vi "OCUMain.vi"() -> ()   [LabVIEW 2014]
uses:
  Command.ctl
  DataHighway.ctl
  <vilib>/Math Plots/2D Math Plots/2D Compass/2D Compass XCtrl/2D Compass.xctl
  MDF.ctl
  <vilib>/Math Plots/2D Math Plots/2D Compass/2D Compass Datatype/Public/Plot Helper (Vector).vi
  <vilib>/ErrorRing/Error Ring.xnode
  <vilib>/Math Plots/2D Math Plots/2D Compass/2D Compass Datatype/2D Compass Datatype.lvclass
panel:
  out "Tug GPS":cluster{"X pos":i32, "Y pos":i32, "Heading":dbl}
  out "UDP Time Out?":bool
  in  "Tug ?":string="T"
  out "Buoy Locations":cluster{"regular expression":string, i32, i32}[](array[cluster])
  out "GPS OK?":bool
  out "Mission Map In":picture
  in  "Stop OCU Code Running":bool
  in  "E-Stop Motors":bool=TRUE
  out "DataHWay":T1
  out "ComHWay":T2 {"Speed" scale=-2.0..10.0; "Rudder" scale=-10.0..10.0}
  out "OCU Running":bool
  out "Tab Control":T3(tab)
  out "PT Mid":dbl(slide) scale=60.0..20.0
  out "ST Mid":dbl(slide) scale=20.0..60.0
  out "ST Bow":dbl(slide) scale=20.0..60.0
  out "Starboard":dbl(slide) scale=20.0..60.0
  out "PT Bow":dbl(slide) scale=20.0..60.0
  out "Boolean 5":bool
  out "Boolean 4":bool
  out "Boolean 3":bool
  out "Boolean 2":bool
  out "Boolean":bool
  in  "Beh Lights ok?":bool
  in  "myRIO ok?":bool
  in  "Prop ok?":bool
  in  "Rudder ok?":bool
  in  "Sharp IR-Lidar ok?":bool
  in  "Goto Debug?":bool
  out "MyRIO":bool
  out "Port":dbl(slide) scale=60.0..20.0
  out "Tug GPS":cluster{"X pos":i32, "Y pos":i32, "Heading":dbl}
  out "Buoy locations":cluster{"regular expression":string, i32, i32}[](array[cluster])
  out "Waiting for Input":bool
  in  "Plan Mission":bool
  in  "Re-Initialize":bool
  in  "Debug Robot":bool
  in  "Run Robot":bool
  in  "Stop OCU":bool
  in  "Prop Speed":dbl(knob)=0.07590623483784206 scale=0.05..0.1
  in  "Rudder":dbl(knob)=0.0742658968653541 scale=0.05..0.1
  in  "Debug Complete?":bool
  out "RobotRunning":bool
  out "HW-Stop":bool
  out "IR LIDAR":refnum<class "2D Plot Datatype.lvclass">[](xcontrol)
  out "Tug GPS Debug":cluster{"X pos":i32, "Y pos":i32, "Heading":dbl}
  out "Buoy Locations Debug":cluster{"regular expression":string, i32, i32}[](array[cluster])
  in  "Exit Run":bool
  out "Tug GPS Run":cluster{"X pos":i32, "Y pos":i32, "Heading":dbl}
  out "Buoy Locations Run":cluster{"regular expression":string, i32, i32}[](array[cluster])
  out "Mission Map Run Robot":picture
  in  "Exit Planning":bool
  in  "Select Behavior":T4(ring)
  out "MDF":T5
  in  "Velocity":dbl(slide) scale=0.0..500.0
  in  "Dwell Time (sec)":dbl(slide) scale=0.0..10.0
  out "Draw Path":bool
  out "WPindex":i32
  in  "Reset MDF":bool
  out "Mission Map":picture
  # "Press Arrow\nabove to start\nOCU running"
  # "Set Tug\nLetter"
  # "G\nT\nL\n?"
  # "Data Highway carries all robot data"
  # "Look at boat. Rudder Oscillating?"
  # "Release E-Stop to test"
  # "Look at boat? Prop Oscillating?"
  # "Is battery attached?"
  # "Look at boat. See Red-Blue-Green?"
  # "Unit Test"
  # "Function"
  # "Run auto Initialize sequence.\nIndicate which functionality is ok.\nAll functions must work or\n choose go to debug state."
  # "Robot Initialized and \nwaiting for user input"
  # "Press button to\nselect robot state"
  # "0.075 rudder center"
  # "0.075 prop off"
  # "OCU and Robot safely shut down"
  # "2. Click on Map to select Waypoints, hold button down and drag to draw tracklines.\n3. Reset MDF and try again if you want to redo your MDF"
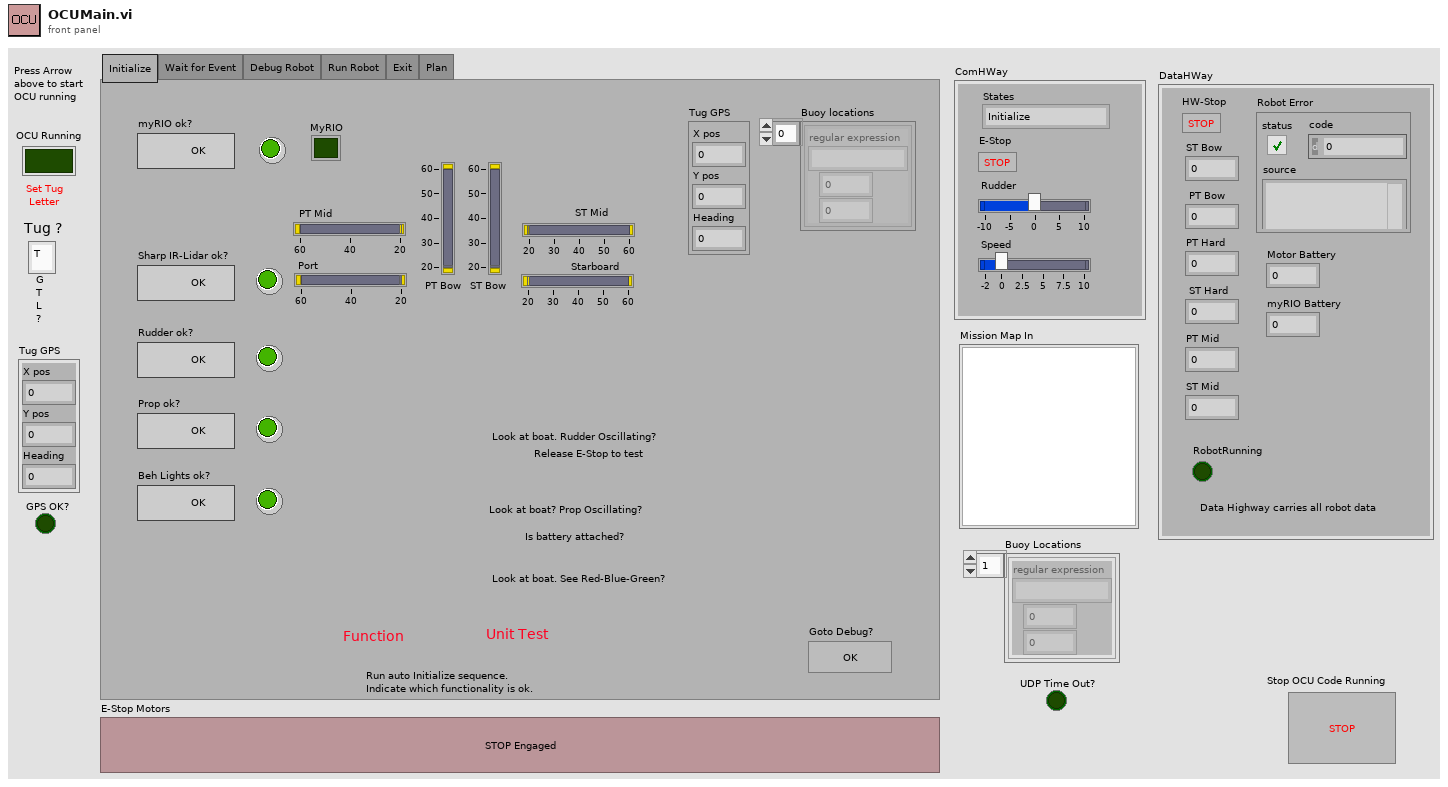
[diagram p1: front panel]
types:
  T1 = typedef "DataHighway.ctl" = cluster{"HW-Stop":bool, "ST Bow":dbl, " PT Bow":dbl, "PT Hard":dbl, "RobotRunning":bool, "Robot Error":errorcluster, " ST Hard":dbl, "PT Mid":dbl, "ST Mid":dbl, "Motor Battery":dbl, "myRIO Battery":dbl}
  T2 = typedef "Command.ctl" = cluster{"States":enum16{"Initialize", "Wait for Event", "Debug Robot", "Run Robot", "Exit", "Plan"}, "E-Stop":bool, "Rudder":dbl, "Speed":dbl}
  T3 = enum32{"Initialize", "Wait for Event", "Debug Robot", "Run Robot", "Exit", "Plan"}
  T4 = enum16{"Stop", "GoToWayPoint", "RightWallFollow", "LeftWallFolllow", "LaneFollow", "CirclePoint"}
  T5 = typedef "MDF.ctl" = cluster{"Status":enum16{"Past", "Current", "Future"}, "x":dbl, "y":dbl, "z":dbl, "Vel":dbl, "Dwell Time":dbl, "BehCom":enum16{"Stop", "GoToWayPoint", "RightWallFollow", "LeftWallFolllow", "LaneFollow", "CirclePoint"}, "Expand1":dbl, "Expand2":dbl, "Expand3":dbl}[]
  T6 = cluster{"Status":enum16{"Past", "Current", "Future"}, "x":dbl, "y":dbl, "z":dbl, "Vel":dbl, "Dwell Time":dbl, "BehCom":enum16{"Stop", "GoToWayPoint", "RightWallFollow", "LeftWallFolllow", "LaneFollow", "CirclePoint"}, "Expand1":dbl, "Expand2":dbl, "Expand3":dbl}
  T7 = enum16{"Initialize", "Wait for Event", "Debug Robot", "Run Robot", "Exit", "Plan"}
  T8 = enum16{"Initialize", "Wait for Event", "Debug Robot", "Run Robot", "Exit"}
  T9 = cluster{"Width":u16, "Style":enum32{"Solid", "Dash", "Dot", "DashDot", "DashDotDot"}}
  T10 = typedef "LVMouseTypeDef.ctl" = cluster{"Mouse Position":cluster{"X":i32, "Y":i32}, "Mouse Modifiers":cluster{"Button Down":bool, "Shift Mod":bool, "Menu Mod":bool, "Option Mod":bool}}
  T11 = cluster{"regular expression":string, i32, i32, i32}
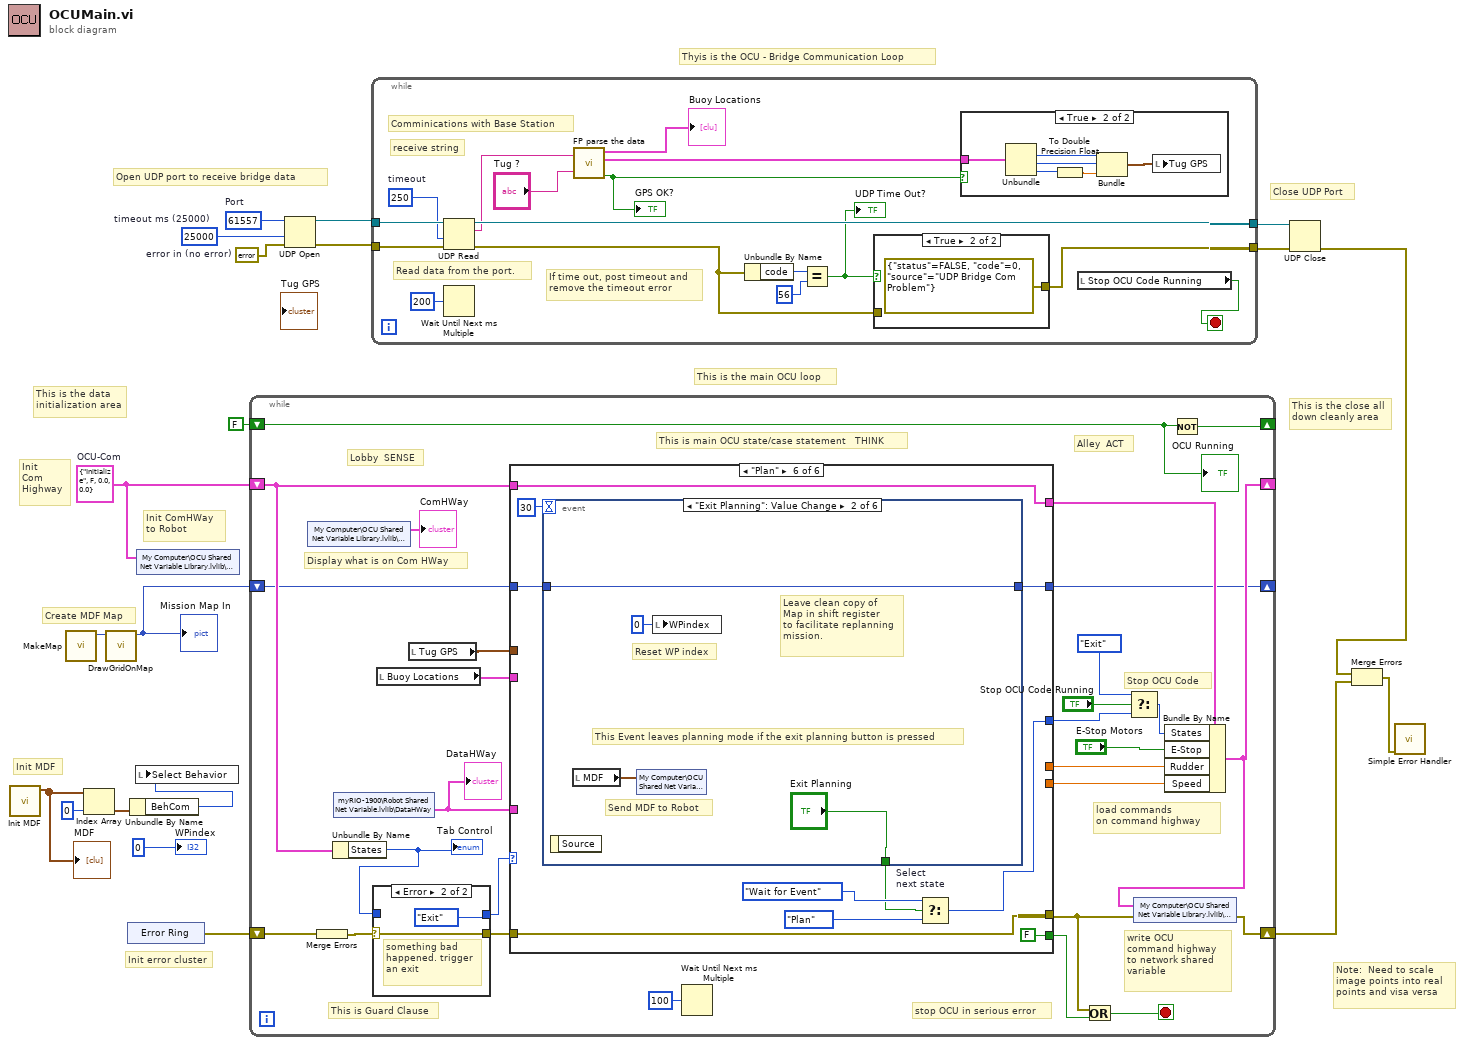
[diagram p0: block diagram]
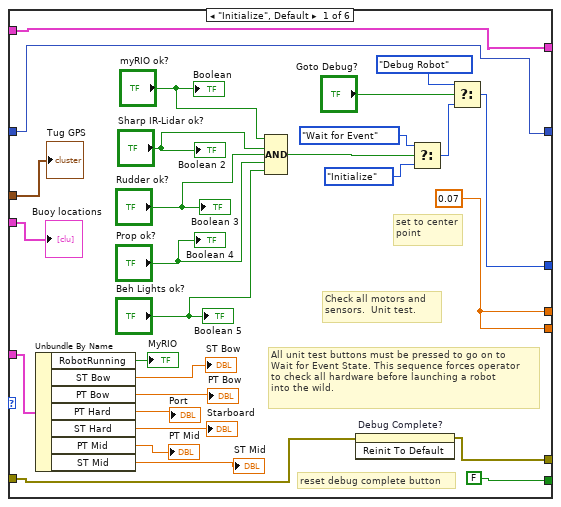
[diagram p5: hidden frame]
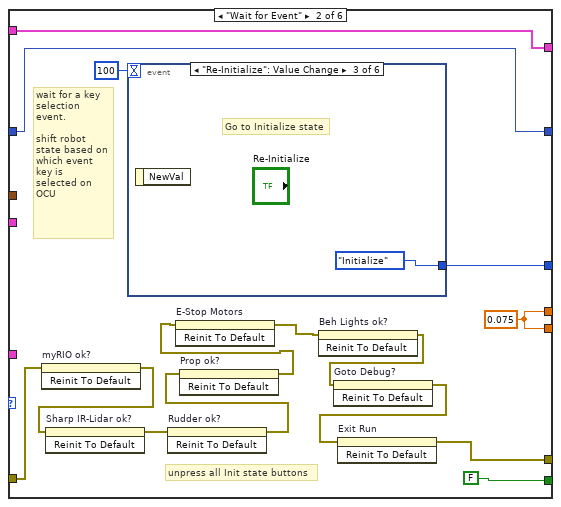
[diagram p6: hidden frame]
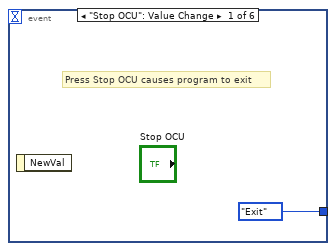
[diagram p7: hidden frame]
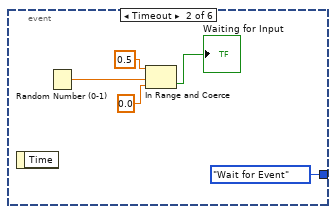
[diagram p8: hidden frame]
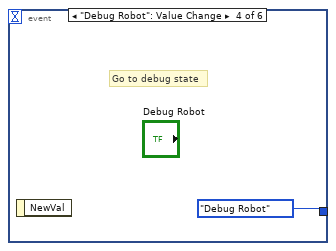
[diagram p9: hidden frame]
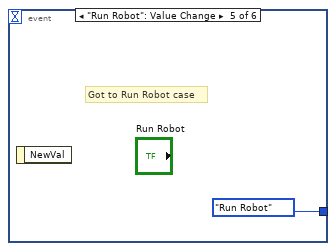
[diagram p10: hidden frame]
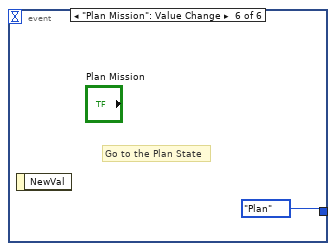
[diagram p11: hidden frame]
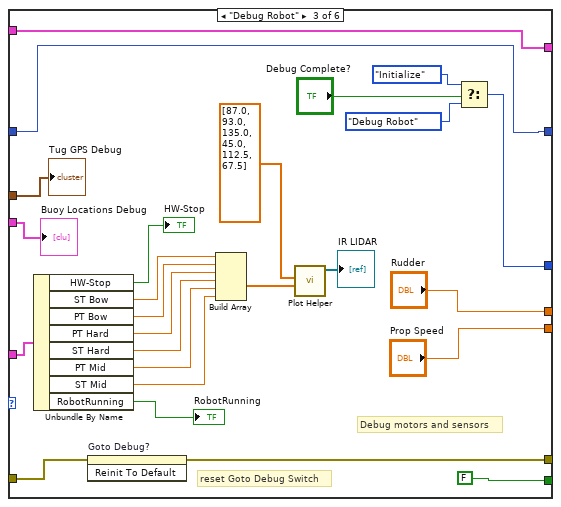
[diagram p12: hidden frame]
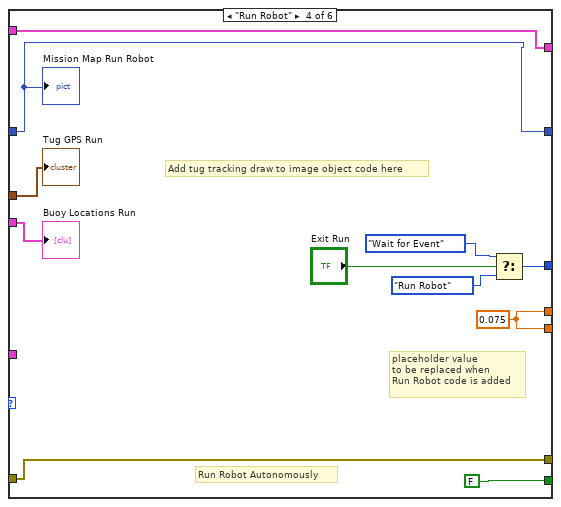
[diagram p13: hidden frame]
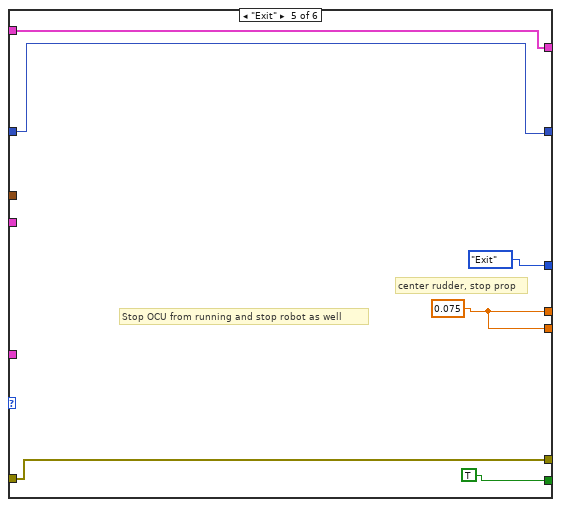
[diagram p14: hidden frame]
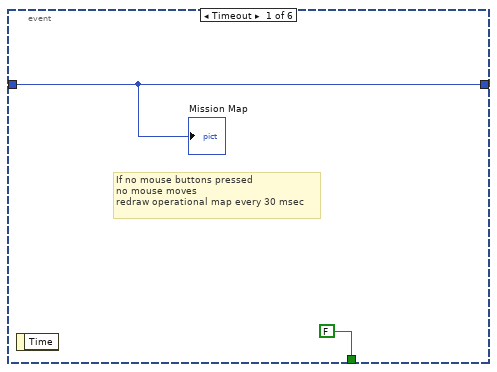
[diagram p15: hidden frame]
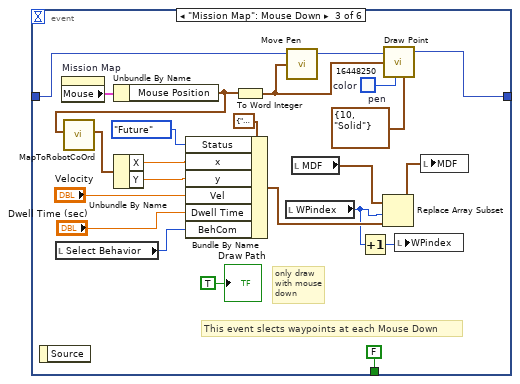
[diagram p16: hidden frame]
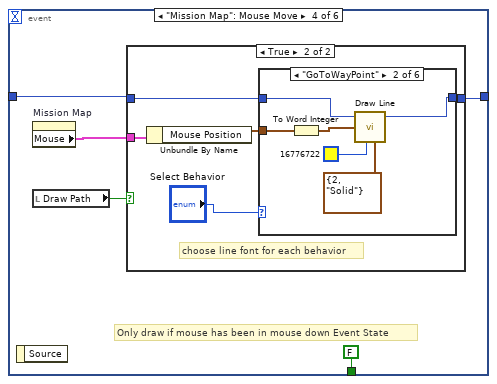
[diagram p17: hidden frame]
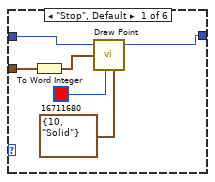
[diagram p19: hidden frame]
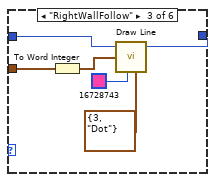
[diagram p20: hidden frame]
diagram:
  w11 = errorcluster {"status"=FALSE, "code"=0, "source"=""}  # error in (no error)
  w9 = 25000  # timeout ms (25000)
  w10 = u16 61557  # Port
  w1 = T2 {"States"=enum."Initialize", "E-Stop"=FALSE, "Rudder"=0.0, "Speed"=0.0}  # OCU-Com
  # "Thyis is the OCU - Bridge Communication Loop"
  # "Close UDP Port"
  # "Create MDF Map"
  # "Open UDP port to receive bridge data"
  # "Note:  Need to scale\nimage points into real \npoints and visa versa"
  # "Init MDF"
  # "Init ComHWay\nto Robot"
  # "Init error cluster"
  # "Init\nCom\nHighway"
  # "This is the close all\ndown cleanly area"
  # "This is the data\ninitialization area"
  # "This is the main OCU loop"
  n1 = call "Init MDF.vi"() -> ("MDF-Out"=w18:T5)  [unwired: 11 in]
  "MDF" <- w18
  n2 = call "MakeMap.vi"() -> ("Operational Map"=w14:picture)  [unwired: 10 in, 1 out]
  n3 = Index Array "Index Array"(array=w18, index=0) -> (element=w16:T6)
  n4 = call "DrawGridOnMap.vi"("Mission MapIn"=w14) -> ("Mission MapOut"=w13:picture)  [unwired: 10 in]
  "Mission Map In" <- w13
  n5 = xnode "Error Ring"() -> ("error out"=w19:errorcluster)
  n6 = Unbundle By Name(w16) -> ("BehCom"=w15:T4)
  n7 = local write "Select Behavior"(w15) -> ()
  n8 = shared-variable "My Computer\\OCU Shared Net Variable Library.lvlib\\ComHWay"(w1) -> ()  [unwired: 1 in, 1 out]
  n9 = while {
    shift-right: [w47] -> _
    shift-left: FALSE -> [w46]
    shift-right: [w39] -> w4
    shift-left: w19 -> [w24]
    shift-right: [w35] -> _
    shift-left: w1 -> [w42]
    shift-right: [w25] -> _
    shift-left: w13 -> [w26]
    stop <- w31 stop-if-true
    # "Stop OCU Code"
    # "load commands\non command highway"
    # "Display what is on Com HWay"
    # "write OCU  \ncommand highway\nto network shared\nvariable"
    # "stop OCU in serious error"
    # "This is Guard Clause"
    # "This is main OCU state/case statement   THINK"
    # "Alley  ACT"
    # "Lobby  SENSE"
    n10 = shared-variable "My Computer\\OCU Shared Net Variable Library.lvlib\\ComHWay"() -> (→"ComHWay":T2)  [unwired: 1 in, 1 out]
    n11 = Merge Errors(w24) -> (w23:errorcluster)
    n12 = Unbundle By Name "Unbundle By Name"(w42) -> ("States"=w41:T7)
    "Tab Control" <- w41
    n13 = shared-variable "myRIO-1900\\Robot Shared Net Variable.lvlib\\DataHWay"() -> (w34:T1)  [unwired: 1 in, 1 out]
    "DataHWay" <- w34
    n14 = case shown="Error" w23 {
      selector: w23 -> [w50 w52]
      tunnel: [w50 w52] -> w45
      tunnel: w41 -> [w49 _]
      tunnel: [w49 T8."Exit" ("States")] -> w43
      frame No Error {
      }
      frame Error {
        # "something bad\nhappened. trigger\nan exit"
      }
    }
    n15 = local read "Buoy Locations"() -> (w21:cluster{"regular expression":string, i32, i32}[])
    n16 = local read "Tug GPS"() -> (w22:cluster{"X pos":i32, "Y pos":i32, "Heading":dbl})
    n17 = case shown="\"Plan\"" w43 {
      tunnel: [w79 w94 w128 w139 T7."Exit" ("States") w148] -> w29
      tunnel: [FALSE FALSE FALSE FALSE TRUE FALSE] -> w44
      tunnel: w45 -> [w62 w93 w125 w137 w146 w157]
      tunnel: [w67 w86 w120 w137 w146 w157] -> w40
      tunnel: w42 -> [w63 w88 w124 w135 w145 w155]
      tunnel: [w63 w88 w124 w135 w145 w155] -> w38
      tunnel: w34 -> [w66 _ w118 _ _ _]
      tunnel: [w64 w85 "Rudder" w134 w144 _] -> w33
      tunnel: [w64 w85 "Prop Speed" w134 w144 _] -> w32
      tunnel: w26 -> [w55 w82 w109 w131 w142 w151]
      tunnel: [w55 w82 w109 w131 w142 w150] -> w25
      tunnel: w22 -> [w54 _ w107 w133 _ _]
      tunnel: w21 -> [w53 _ w106 w132 _ _]
      frame "Initialize", Default {
        w64 = 0.07 ("Rudder")
        # "set to center\npoint"
        # "reset debug complete button"
        # "All unit test buttons must be pressed to go on to \nWait for Event State. This sequence forces operator\nto check all hardware before launching a robot\ninto the wild."
        # "Check all motors and \nsensors.  Unit test."
        n18 = Unbundle By Name(w66) -> ("RobotRunning"=→"MyRIO":bool, "ST Bow"=→"ST Bow":dbl, "PT Bow"=→"PT Bow":dbl, "PT Hard"=→"Port":dbl, "ST Hard"=→"Starboard":dbl, "PT Mid"=→"PT Mid":dbl, "ST Mid"=→"ST Mid":dbl)
        n19 = Compound Arithmetic op=AND("myRIO ok?", "Sharp IR-Lidar ok?", "Rudder ok?", "Prop ok?", "Beh Lights ok?") -> (w68:bool)
        n20 = invoke on="Debug Complete?" class="Bool (strict)" method="Reinit To Default"(error in=w62) -> (error out=w67:errorcluster)  [unwired: 2 in, 2 out]
        n21 = Select ("Select next state")(t=T8."Wait for Event" ("States"), s=w68, f=T8."Initialize") -> (s? t:f=w76:T8)
        n22 = Select ("Select next state")(t=T8."Debug Robot" ("f"), s="Goto Debug?", f=w76) -> (s? t:f=w79:T8)
        "Boolean" <- "myRIO ok?"
        "Boolean 2" <- "Sharp IR-Lidar ok?"
        "Boolean 3" <- "Rudder ok?"
        "Boolean 4" <- "Prop ok?"
        "Boolean 5" <- "Beh Lights ok?"
        "Tug GPS" <- w54
        "Buoy locations" <- w53
      }
      frame "Wait for Event" {
        w85 = 0.075 ("Rudder")
        # "unpress all Init state buttons"
        # "wait for a key \nselection\nevent.\n\nshift robot\nstate based on\nwhich event\nkey is\nselected on \nOCU"
        n23 = invoke on="myRIO ok?" class="Bool (strict)" method="Reinit To Default"(error in=w93) -> (error out=w92:errorcluster)  [unwired: 2 in, 2 out]
        n24 = invoke on="Sharp IR-Lidar ok?" class="Bool (strict)" method="Reinit To Default"(error in=w92) -> (error out=w91:errorcluster)  [unwired: 2 in, 2 out]
        n25 = event shown="[2] \"Re-Initialize\": Value Change" {
          selector: _ -> [_ _ _ _ _ _]
          dyn-events: _ -> [_ _ _ _ _ _]
          timeout: 100 -> [_ _ _ _ _ _]
          tunnel: [T7."Exit" ("States") T7."Wait for Event" ("States") T7."Initialize" ("States") T7."Debug Robot" ("States") T7."Run Robot" ("States") T7."Plan" ("States")] -> w94
          event "Stop OCU": Value Change {
            # "Press Stop OCU causes program to exit"
            n26 = event-data() -> ()  [unwired: 1 in, 1 out]
          }
          event Timeout {
            n27 = event-data() -> ()  [unwired: 1 in, 1 out]
            n28 = Random Number (0-1)() -> (number: 0 to 1=w100:dbl)
            n29 = In Range and Coerce(upper limit=0.5, x=w100, lower limit=0.0) -> (In Range?=→"Waiting for Input":bool)  [unwired: 1 out]
          }
          event "Re-Initialize": Value Change {
            # "Go to Initialize state"
            n30 = event-data() -> ()  [unwired: 1 in, 1 out]
          }
          event "Debug Robot": Value Change {
            # "Go to debug state"
            n31 = event-data() -> ()  [unwired: 1 in, 1 out]
          }
          event "Run Robot": Value Change {
            # "Got to Run Robot case"
            n32 = event-data() -> ()  [unwired: 1 in, 1 out]
          }
          event "Plan Mission": Value Change {
            # "Go to the Plan State"
            n33 = event-data() -> ()  [unwired: 1 in, 1 out]
          }
        }
        n34 = invoke on="Rudder ok?" class="Bool (strict)" method="Reinit To Default"(error in=w91) -> (error out=w90:errorcluster)  [unwired: 2 in, 2 out]
        n35 = invoke on="Prop ok?" class="Bool (strict)" method="Reinit To Default"(error in=w90) -> (error out=w84:errorcluster)  [unwired: 2 in, 2 out]
        n36 = invoke on="E-Stop Motors" class="Bool (strict)" method="Reinit To Default"(error in=w84) -> (error out=w83:errorcluster)  [unwired: 2 in, 2 out]
        n37 = invoke on="Beh Lights ok?" class="Bool (strict)" method="Reinit To Default"(error in=w83) -> (error out=w89:errorcluster)  [unwired: 2 in, 2 out]
        n38 = invoke on="Goto Debug?" class="Bool (strict)" method="Reinit To Default"(error in=w89) -> (error out=w87:errorcluster)  [unwired: 2 in, 2 out]
        n39 = invoke on="Exit Run" class="Bool (strict)" method="Reinit To Default"(error in=w87) -> (error out=w86:errorcluster)  [unwired: 2 in, 2 out]
      }
      frame "Debug Robot" {
        # "reset Goto Debug Switch"
        # "Debug motors and sensors"
        n40 = Unbundle By Name "Unbundle By Name"(w118) -> ("HW-Stop"=→"HW-Stop":bool, "ST Bow"=w108:dbl, "PT Bow"=w116:dbl, "PT Hard"=w115:dbl, "ST Hard"=w114:dbl, "PT Mid"=w113:dbl, "ST Mid"=w112:dbl, "RobotRunning"=→"RobotRunning":bool)
        n41 = invoke on="Goto Debug?" class="Bool (strict)" method="Reinit To Default"(error in=w125) -> (error out=w120:errorcluster)  [unwired: 2 in, 2 out]
        n42 = Build Array "Build Array"(w108, w116, w115, w114, w113, w112) -> (w111:dbl[])
        n43 = call-poly <vilib>:"Plot Helper.vi"("radius vector"=w111, "theta vector"=dbl[] [87.0, 93.0, 135.0, 45.0, 112.5, 67.5]) -> ("2D Plot Class Obj Array out"=→"IR LIDAR":refnum<class "2D Plot Datatype.lvclass">[])  [unwired: 2 in, 7 out]
        n44 = Select(t=T8."Initialize" ("States"), s="Debug Complete?", f=T8."Debug Robot") -> (s? t:f=w128:T8)
        "Tug GPS Debug" <- w107
        "Buoy Locations Debug" <- w106
      }
      frame "Run Robot" {
        w134 = 0.075 ("Rudder")
        # "Add tug tracking draw to image object code here"
        # "placeholder value\nto be replaced when \nRun Robot code is added"
        # "Run Robot Autonomously"
        n45 = Select(t=T8."Wait for Event" ("States"), s="Exit Run", f=T8."Run Robot") -> (s? t:f=w139:T8)
        "Tug GPS Run" <- w133
        "Buoy Locations Run" <- w132
        "Mission Map Run Robot" <- w131
      }
      frame "Exit" {
        w144 = 0.075 ("Rudder")
        # "center rudder, stop prop"
        # "Stop OCU from running and stop robot as well"
      }
      frame "Plan" {
        n46 = event shown="[1] \"Exit Planning\": Value Change" {
          selector: _ -> [_ _ _ _ _ _]
          dyn-events: _ -> [_ _ _ _ _ _]
          timeout: 30 -> [_ _ _ _ _ _]
          tunnel: w151 -> [w159 w162 w186 w191 w236 _]
          tunnel: [w159 w162 w182 w190 w236 w238] -> w150
          tunnel: [FALSE "Exit Planning" FALSE ("Exit Planning") FALSE ("Exit Planning") FALSE ("Exit Planning") FALSE ("Exit Planning")] -> w149
          event Timeout {
            # "If no mouse buttons pressed\nno mouse moves\nredraw operational map every 30 msec"
            n47 = event-data() -> ()  [unwired: 1 in, 1 out]
            "Mission Map" <- w159
          }
          event "Exit Planning": Value Change {
            # "Send MDF to Robot"
            # "Reset WP index"
            # "This Event leaves planning mode if the exit planning button is pressed"
            # "Leave clean copy of\nMap in shift register\nto facilitate replanning\nmission."
            n48 = event-data() -> ()  [unwired: 1 in, 1 out]
            n49 = local read "MDF"() -> (w160:T5)
            n50 = shared-variable "My Computer\\OCU Shared Net Variable Library.lvlib\\MDF"(w160) -> ()  [unwired: 1 in, 1 out]
            n51 = local write "WPindex"(0 ("WPindex")) -> ()
          }
          event "Mission Map": Mouse Down {
            w183 = T9 {"Width"=10, "Style"=enum."Solid"}  # pen
            w184 = u32 16448250  # color
            # "only draw\nwith mouse \ndown"
            # "This event slects waypoints at each Mouse Down"
            n52 = event-data() -> ()  [unwired: 1 in, 1 out]
            n53 = local read "Select Behavior"() -> (w170:T4)
            n54 = property on="Mission Map" class="Pict"() -> ("Mouse"=w181:T10)  [unwired: 2 in, 2 out]
            n55 = Unbundle By Name(w181) -> ("Mouse Position"=w179:cluster{"X":i32, "Y":i32})
            n56 = call "MapToRobotCoOrd.vi"("WP Map"=w179) -> ("WP Robot"=w178:cluster{"X":dbl, "Y":dbl})  [unwired: 10 in]
            n57 = Unbundle By Name(w178) -> ("X"=w175:dbl, "Y"=w174:dbl)
            n58 = Bundle By Name(cluster=T6 {"Status"=enum."Past", "x"=0.0, "y"=0.0, "z"=0.0, "Vel"=0.0, "Dwell Time"=0.0, "BehCom"=enum."Stop", "Expand1"=0.0, "Expand2"=0.0, "Expand3"=0.0} ("MissionDefinitionFile"), "Status"=enum16{"Past", "Current", "Future"}."Future", "x"=w175, "y"=w174, "Vel"="Velocity", "Dwell Time"="Dwell Time (sec)", "BehCom"=w170) -> (w167:T6)
            n59 = To Word Integer(number=w179) -> (16bit integer=w180:cluster{"X":i16, "Y":i16})
            n60 = local read "WPindex"() -> (w165:i32)
            n61 = call <vilib>:"Move Pen.vi"("new position"=w180, "picture"=w186) -> ("new picture"=w185:picture)  [unwired: 3 in]
            n62 = local read "MDF"() -> (w169:T5)
            n63 = Increment(x=w165) -> (x+1=w166:i32)
            n64 = Replace Array Subset "Replace Array Subset"(array=w169, new element=w167, index=w165) -> (w168:T5)
            n65 = call <vilib>:"Draw Point.vi"("picture"=w185, "point(x,y)"=w180, "color(black)"=w184, "pen"=w183) -> ("new picture"=w182:picture)  [unwired: 5 in]
            n66 = local write "WPindex"(w166) -> ()
            n67 = local write "MDF"(w168) -> ()
            "Draw Path" <- TRUE ("Draw Path")
          }
          event "Mission Map": Mouse Move {
            # "Only draw if mouse has been in mouse down Event State"
            n68 = event-data() -> ()  [unwired: 1 in, 1 out]
            n69 = property on="Mission Map" class="Pict"() -> ("Mouse"=w188:T10)  [unwired: 2 in, 2 out]
            n70 = local read "Draw Path"() -> (w187:bool)
            n71 = case shown="True" w187 {
              tunnel: w191 -> [w192 w197]
              tunnel: [w192 w196] -> w190
              tunnel: w188 -> [_ w195]
              frame False {
                # "Mouse button not down.\nDrawPath set to false.\nDon't Draw."
              }
              frame True {
                # "choose line font for each behavior"
                n72 = Unbundle By Name "Unbundle By Name"(w195) -> ("Mouse Position"=w194:cluster{"X":i32, "Y":i32})
                n73 = case shown="\"GoToWayPoint\"" "Select Behavior" {
                  tunnel: w197 -> [w203 w209 w213 w219 w225 w233]
                  tunnel: [w202 w208 w212 w218 w224 w232] -> w196
                  tunnel: w194 -> [w201 w207 w211 w217 w223 w229]
                  frame "Stop", Default {
                    n74 = To Word Integer(number=w201) -> (16bit integer=w198:cluster{"X":i16, "Y":i16})
                    n75 = call <vilib>:"Draw Point.vi"("picture"=w203, "point(x,y)"=w198, "color(black)"=u32 16711680, "pen"=T9 {"Width"=10, "Style"=enum."Solid"}) -> ("new picture"=w202:picture)  [unwired: 5 in]
                  }
                  frame "GoToWayPoint" {
                    n76 = To Word Integer(number=w207) -> (16bit integer=w206:cluster{"X":i16, "Y":i16})
                    n77 = call <vilib>:"Draw Line.vi"("picture"=w209, "end point"=w206, "color(black)"=u32 16776722, "pen"=T9 {"Width"=2, "Style"=enum."Solid"}) -> ("new picture"=w208:picture)  [unwired: 5 in]
                  }
                  frame "RightWallFollow" {
                    n78 = To Word Integer(number=w211) -> (16bit integer=w210:cluster{"X":i16, "Y":i16})
                    n79 = call <vilib>:"Draw Line.vi"("picture"=w213, "end point"=w210, "color(black)"=u32 16728743, "pen"=T9 {"Width"=3, "Style"=enum."Dot"}) -> ("new picture"=w212:picture)  [unwired: 5 in]
                  }
                  frame "LeftWallFolllow" {
                    n80 = To Word Integer(number=w217) -> (16bit integer=w216:cluster{"X":i16, "Y":i16})
                    n81 = call <vilib>:"Draw Line.vi"("picture"=w219, "end point"=w216, "color(black)"=u32 1245167, "pen"=T9 {"Width"=3, "Style"=enum."Dot"}) -> ("new picture"=w218:picture)  [unwired: 5 in]
                  }
                  frame "LaneFollow" {
                    n82 = To Word Integer(number=w223) -> (16bit integer=w222:cluster{"X":i16, "Y":i16})
                    n83 = call <vilib>:"Draw Line.vi"("picture"=w225, "end point"=w222, "color(black)"=u32 16757546, "pen"=T9 {"Width"=3, "Style"=enum."Dash"}) -> ("new picture"=w224:picture)  [unwired: 5 in]
                  }
                  frame "CirclePoint" {
                    n84 = To Word Integer(number=w229) -> (16bit integer=w228:cluster{"X":i16, "Y":i16})
                    n85 = call <vilib>:"Draw Point.vi"("picture"=w233, "point(x,y)"=w228, "color(black)"=u32 16748288, "pen"=T9 {"Width"=20, "Style"=enum."Solid"}) -> ("new picture"=w232:picture)  [unwired: 5 in]
                  }
                }
              }
            }
          }
          event "Mission Map": Mouse Up {
            # "Finish drawing WP path when mouse button is let up.\nSet Draw Path to False."
            n86 = event-data() -> ()  [unwired: 1 in, 1 out]
            n87 = local write "Draw Path"(FALSE ("Draw Path")) -> ()
          }
          event "Reset MDF": Value Change {
            # "Event \nresets map\nabd MDF"
            # "Redraw map with clean new copy"
            n88 = event-data() -> ()  [unwired: 1 in, 1 out]
            n89 = for {
              N: 25 -> [_]
              i -> [w242]
              # "This event reinitializes\nthe MDF array with the\nvalues shown to the left"
              n90 = local read "MDF"() -> (w241:T5)
              n91 = Replace Array Subset(array=w241, new element=T6 {"Status"=enum."Future", "x"=0.0, "y"=0.0, "z"=0.0, "Vel"=0.0, "Dwell Time"=0.0, "BehCom"=enum."Stop", "Expand1"=0.0, "Expand2"=0.0, "Expand3"=0.0} ("new element/subarray"), index=w242) -> (w240:T5)
              n92 = local write "MDF"(w240) -> ()
            }
            n93 = local read "Mission Map In"() -> (w238:picture)
          }
        }
        n94 = Select "Select \nnext state"(t=T7."Wait for Event" ("States"), s=w149, f=T7."Plan" ("States")) -> (s? t:f=w148:T7)
      }
    }
    n95 = Wait Until Next ms Multiple(millisecond multiple=u32 100) -> ()  [unwired: 1 out]
    n96 = Or(x=w40, y=w44) -> (x .or. y?=w31:bool)
    n97 = Select(t=T7."Exit" ("States"), s="Stop OCU Code Running", f=w29) -> (s? t:f=w28:T7)
    n98 = Bundle By Name(cluster=w38, "States"=w28, "E-Stop"="E-Stop Motors", "Rudder"=w33, "Speed"=w32) -> (w35:T2)
    n99 = shared-variable "My Computer\\OCU Shared Net Variable Library.lvlib\\ComHWay"(w35, error in=w40) -> (error out=w39:errorcluster)
    n100 = Not(x=w46) -> (.not. x?=w47:bool)
    "OCU Running" <- w46
  }
  n101 = UDP Open(8:w11, 9:w9, 11:w10) -> (port=w8:refnum<k16>, 0:w5:errorcluster)  [unwired: 2 in, 1 out]
  n102 = while {
    tunnel: w5 -> [w259]
    tunnel: w8 -> [w258]
    tunnel: [w257] -> w7
    tunnel: [w252] -> w6
    stop <- w244 stop-if-true
    w251 = 250  # timeout
    # "Comminications with Base Station"
    # "receive string"
    # "If time out, post timeout and\nremove the timeout error"
    # "Read data from the port."
    n103 = UDP Read(connection ID=w258, timeout ms (25000)=w251, 8:w259) -> (data out=w247:string, error out=w253:errorcluster, 3:w257:refnum<k16>)  [unwired: 1 in, 2 out]
    n104 = Wait Until Next ms Multiple(millisecond multiple=u32 200) -> ()  [unwired: 1 out]
    n105 = call "FP parse the data.vi"("Nav String"=w247, "Tug"="Tug ?") -> ("Buoy locations"=→"Buoy Locations":cluster{"regular expression":string, i32, i32}[], "Tug Location"=w248:T11, "Valid?"=w245:bool)  [unwired: 1 out]
    "GPS OK?" <- w245
    n106 = Unbundle By Name(w253) -> ("code"=w256:i32)
    n107 = Equal?(x=w256, y=56) -> (x = y?=w254:bool)
    "UDP Time Out?" <- w254
    n108 = case shown="True" w254 {
      tunnel: [w266 errorcluster {"status"=FALSE, "code"=0, "source"="UDP Bridge Com Problem"} ("error out")] -> w252
      tunnel: w253 -> [w266 _]
      frame False {
      }
      frame True {
      }
    }
    n109 = case shown="True" w245 {
      tunnel: w248 -> [_ w265]
      frame False {
      }
      frame True {
        n110 = Unbundle(w265) -> (w264:i32, w263:i32, w261:i32)  [unwired: 1 out]
        n111 = To Double Precision Float(number=w261) -> (double precision float=w262:dbl)
        n112 = Bundle(w264, w263, w262) -> (w260:cluster{i32, i32, dbl})  [unwired: 1 in]
        n113 = local write "Tug GPS"(w260) -> ()
      }
    }
    n114 = local read "Stop OCU Code Running"() -> (w244:bool)
  }
  n115 = UDP Close(connection ID=w7, 8:w6) -> (error out=w2:errorcluster)  [unwired: 1 out]
  n116 = Merge Errors(w2, w4) -> (w3:errorcluster)
  n117 = call <vilib>:"Simple Error Handler.vi"("error in (no error)"=w3) -> ()  [unwired: 4 in, 5 out]
  "WPindex" <- 0 ("WPindex")
